vi "dll.midi_create_manager.vi"(8 "error in (no error)":errorcluster, 11 "midi out in":refnum<class "midi out.lvclass">) -> (0 "error out":errorcluster, 3 "midi out":refnum<class "midi out.lvclass">)   [LabVIEW 2020, in "midi out.lvclass"]
uses:
  midi out.lvclass
  midi out.lvclass/midi out.ctl
  shared/midi shared.lvlib
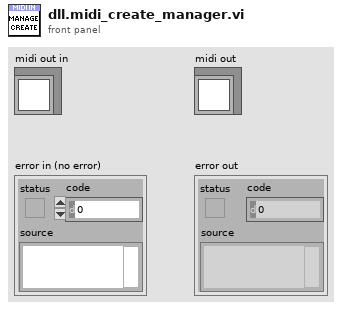
[diagram p1: front panel]
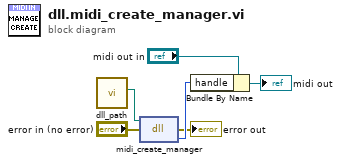
[diagram p0: block diagram]
diagram:
  n1 = call "dll_path.vi"() -> ("dll"=w4:path)  [unwired: 11 in]
  n2 = dll-call lib="C:/code/LabVIEW-MIDI-XPLAT/dist/TomMIDIllan_*.*" fn="midi_create_manager"(path in=w4, error in="error in (no error)") -> (error out=→"error out":errorcluster, "Handle"=w5:i32)  [unwired: 1 in, 1 out]
  n3 = Bundle By Name(cluster="midi out in", "handle"=w5) -> (→"midi out":refnum<class "midi out.lvclass">)
